vi "Get File Version Number.vi"(8 "Error In":errorcluster, 11 "Filepath":path) -> (0 "Error Out":errorcluster, 3 "File Version Number":string)   [LabVIEW 2023, in "Error Manager.lvlib"]
doc: "Retrieves the File Version of a file. This VI calls (and is based on) Win32 API function version.dll:GetFileVersionInfoA ( https://docs.microsoft.com/en-us/windows/win32/api/winver/nf-winver-getfileversioninfoa ).\n\nThis VI can execute only on a Windows target (My Computer)."
uses:
  Error Manager.lvlib
  version.dll
panel:
  out "File Version Size (Number Of Bytes)":u32
  out "Return Value":u8
  out "Return String (unprocessed)":string
  # "Development\ncontrols/indicators useful for development and testing, but which are not outputs of the VI"
  # "Input\nInputs to the VI"
  # "Output\nOutputs of the VI"
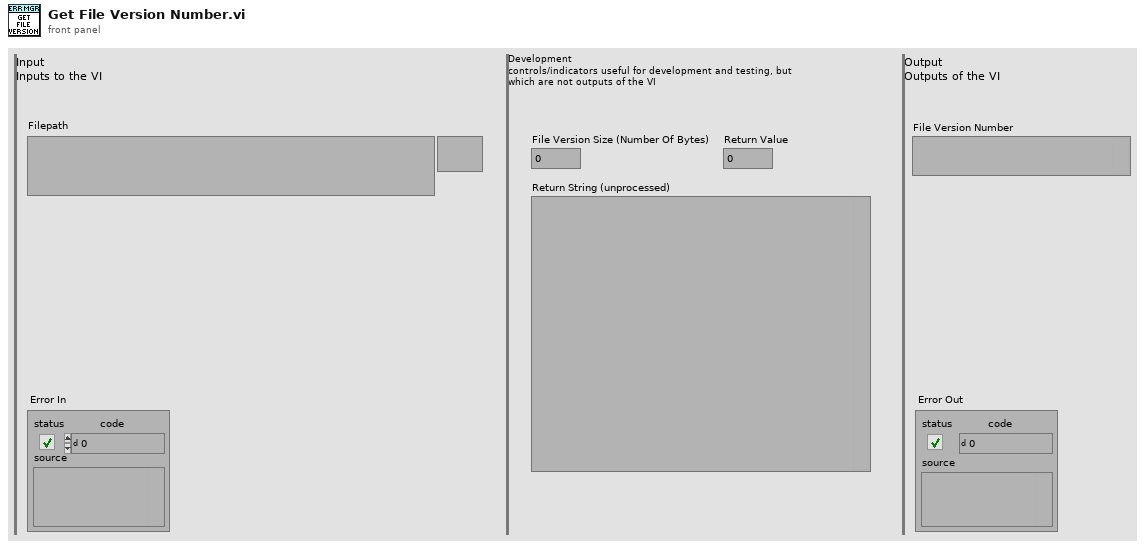
[diagram p1: front panel]
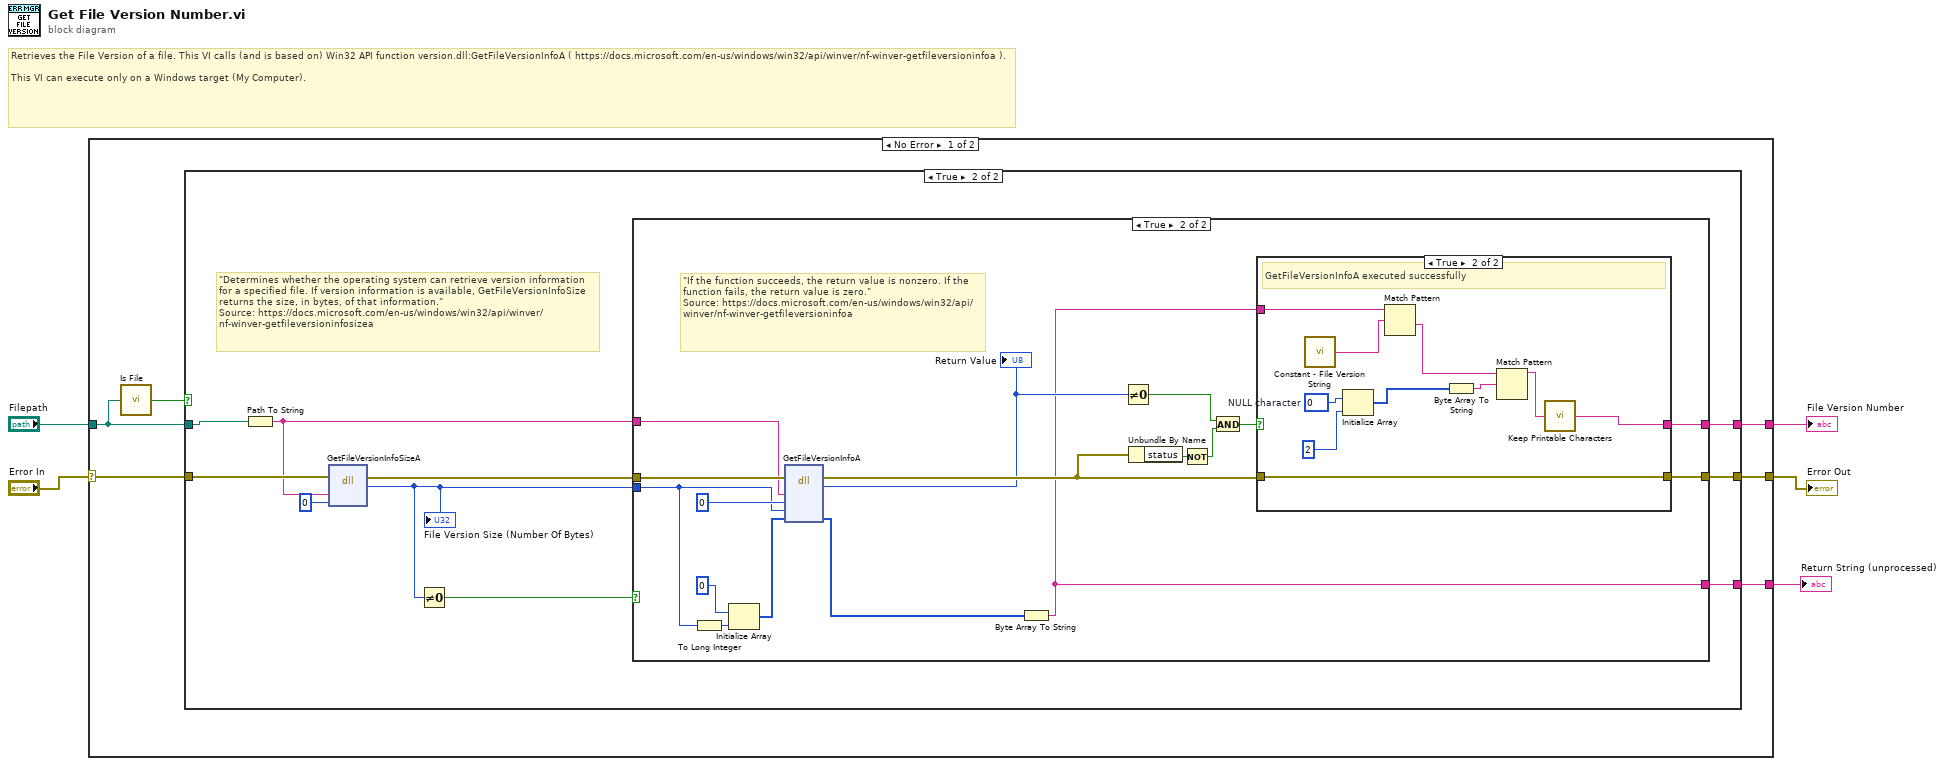
[diagram p0: block diagram]
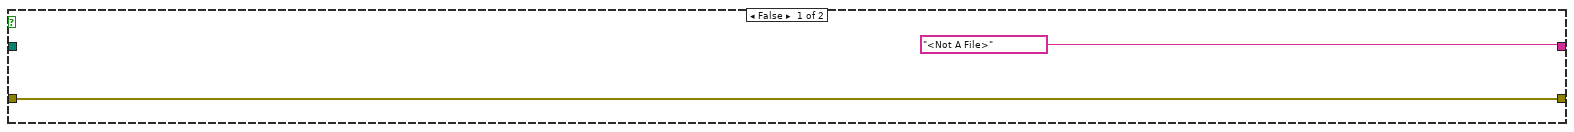
[diagram p2: hidden frame]
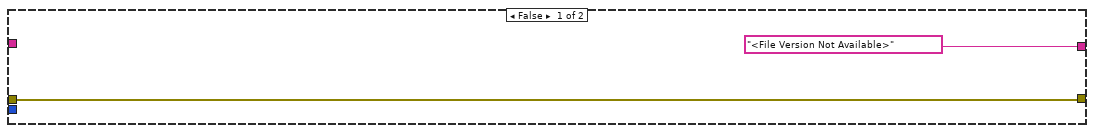
[diagram p3: hidden frame]
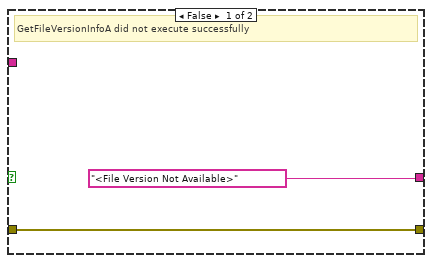
[diagram p4: hidden frame]
diagram:
  # "Retrieves the File Version of a file. This VI calls (and is based on) Win32 API function version.dll:GetFileVersionInfoA ( https://docs.microsoft.com/en-us/windows/win32/api/winver/nf-winver-getfileversioninfoa ).\n\nThis VI can execute only on a Windows target (My Computer)."
  n1 = case shown="No Error" "Error In" {
    selector: "Error In" -> [w11 w55]
    tunnel: [w10 w55] -> w4
    tunnel: [w9 _] -> w3
    tunnel: "Filepath" -> [w8 _]
    tunnel: [w6 _] -> w1
    frame No Error {
      n2 = call "Is File.vi"("Input Path"=w8) -> ("Is Existing File?"=w7:bool)
      n3 = case shown="True" w7 {
        tunnel: w11 -> [w13 w20]
        tunnel: [w13 w23] -> w10
        tunnel: ["<Not A File>" ("pattern label") w22] -> w9
        tunnel: w8 -> [_ w21]
        tunnel: [_ w14] -> w6
        frame False {
        }
        frame True {
          # "\"Determines whether the operating system can retrieve version information for a specified file. If version information is available, GetFileVersionInfoSize returns the size, in bytes, of that information.\"\nSource: https://docs.microsoft.com/en-us/windows/win32/api/winver/nf-winver-getfileversioninfosizea"
          n4 = Path To String(path=w21) -> (string=w18:string)
          n5 = dll-call lib="version.dll" fn="GetFileVersionInfoSizeA"(error in=w20, "lptstrFilename"=w18, "dwHandle"=0) -> (error out=w19:errorcluster, "return type"=w15:u32)  [unwired: 4 in, 1 out]
          "File Version Size (Number Of Bytes)" <- w15
          n6 = Not Equal To 0?(x=w15) -> (x != 0?=w16:bool)
          n7 = case shown="True" w16 {
            tunnel: [w25 w38] -> w23
            tunnel: ["<File Version Not Available>" ("result string") w27] -> w22
            tunnel: w19 -> [w25 w36]
            tunnel: w18 -> [_ w35]
            tunnel: w15 -> [_ w34]
            tunnel: [_ w26] -> w14
            frame False {
            }
            frame True {
              # "\"If the function succeeds, the return value is nonzero. If the function fails, the return value is zero.\"\nSource: https://docs.microsoft.com/en-us/windows/win32/api/winver/nf-winver-getfileversioninfoa"
              n8 = To Long Integer(number=w34) -> (32bit integer=w33:i32)
              n9 = Initialize Array(u8 0 ("element"), w33) -> (w42:u8[])
              n10 = dll-call lib="version.dll" fn="GetFileVersionInfoA"(error in=w36, "lptstrFilename"=w35, "dwHandle"=0, "dwLen"=w34, "lpData"=w42) -> (error out=w39:errorcluster, "return type"=w32:u8, "lpData"=w37:u8[])  [unwired: 5 in, 1 out]
              "Return Value" <- w32
              n11 = Byte Array To String(unsigned byte array=w37) -> (string=w26:string)
              n12 = Not Equal To 0?(x=w32) -> (x != 0?=w31:bool)
              n13 = Unbundle By Name(w39) -> ("status"=w30:bool)
              n14 = Not(x=w30) -> (.not. x?=w29:bool)
              n15 = And(x=w31, y=w29) -> (x .and. y?=w28:bool)
              n16 = case shown="True" w28 {
                tunnel: w39 -> [w44 w54]
                tunnel: [w44 w54] -> w38
                tunnel: w26 -> [_ w53]
                tunnel: ["<File Version Not Available>" ("result string") w52] -> w27
                frame False {
                  # "GetFileVersionInfoA did not execute successfully"
                }
                frame True {
                  w46 = u8 0  # NULL character
                  # "GetFileVersionInfoA executed successfully"
                  n17 = call "Constant - File Version String.vi"() -> ("File Version String (to search for this in output of version.dll:GetFileVersionInfoA)"=w51:string)
                  n18 = Initialize Array(w46, 2 ("dimension size")) -> (w47:u8[])
                  n19 = Match Pattern(string=w53, regular expression=w51) -> (after substring=w45:string)  [unwired: 1 in, 3 out]
                  n20 = Byte Array To String(unsigned byte array=w47) -> (string=w49:string)
                  n21 = Match Pattern(string=w45, regular expression=w49) -> (before substring=w50:string)  [unwired: 1 in, 3 out]
                  n22 = call "Keep Printable Characters.vi"("String in"=w50) -> ("String out (printable characters only - ASCII 0x20 to 0x7F)"=w52:string)
                }
              }
            }
          }
        }
      }
    }
    frame Error {
    }
  }
  "Error Out" <- w4
  "File Version Number" <- w3
  "Return String (unprocessed)" <- w1
